vi "post_new_group.vi"(8 "error in (no error)":errorcluster, 11 "Group Name":string) -> (0 "error out":errorcluster)   [LabVIEW 2013]
doc: "Adds a the given cluster to the pelletron_data table."
uses:
  <vilib>/addons/database/_DB Variant To Data/Database Variant To Data.xnode
  <vilib>/addons/database/NI_Database_API.lvlib
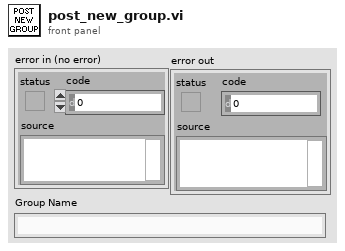
[diagram p1: front panel]
types:
  T1 = typedef "NI_Database_API.lvlib/Conn ObjectReference.ctl" = refnum<k1>
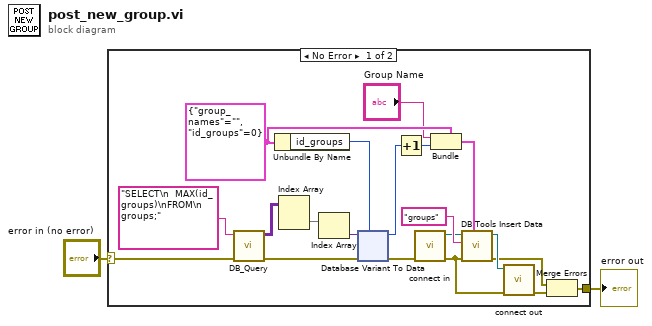
[diagram p0: block diagram]
diagram:
  n1 = case shown="No Error" "error in (no error)" {
    selector: "error in (no error)" -> [w15 w55]
    tunnel: [w16 w55] -> w1
    frame No Error {
      w7 = cluster{"group_names":string, "id_groups":u16} {"group_names"="", "id_groups"=0}
      n2 = call "DB_Query.vi"("error in (no error)"=w15, "Parameterized Query"="SELECT\n  MAX(id_groups)\nFROM\n groups;") -> ("error out"=w13:errorcluster, "Results"=w10:variant[][])  [unwired: 7 in, 1 out]
      n3 = Unbundle By Name(w7) -> ("id_groups"=w11:u16)
      n4 = Index Array(array=w10) -> (element=w9:variant[])  [unwired: 2 in]
      n5 = Index Array(array=w9) -> (element=w8:variant)  [unwired: 1 in]
      n6 = xnode "Database Variant To Data"("database variant"=w8, "error in (no error)"=w13, "type"=w11) -> ("data"=w5:u16, "error out"=w12:errorcluster)
      n7 = Increment(x=w5) -> (x+1=w4:u16)
      n8 = call "connect in.vi"("error in (no error)"=w12) -> ("error out"=w18:errorcluster, "Database Connection"=w21:T1)  [unwired: 7 in]
      n9 = Bundle(cluster=w7, "group_names"="Group Name", "id_groups"=w4) -> (w3:cluster{"group_names":string, "id_groups":u16})
      n10 = call <vilib>:"DB Tools Insert Data.vi"("data"=w3, "error in (no error)"=w18, "table"="groups", "connection reference"=w21) -> ("error out"=w19:errorcluster, "connection reference out"=w20:T1)  [unwired: 6 in]
      n11 = call "connect out.vi"("error in (no error)"=w18, "connection reference"=w20) -> ("error out"=w17:errorcluster)  [unwired: 9 in]
      n12 = Merge Errors(w19, w17) -> (w16:errorcluster)
    }
    frame Error {
    }
  }
  "error out" <- w1
